vi "RUS Sweep -- write line to Temperatures file.vi"(4 "voltage":dbl, 6 "filename cluster OUT":T1={"mmddyy (str)"="", "counter (str)"="", "to F (kHz)"=0.0, "from F (kHz)"=0.0, "temperature (K)"=0.0, "date/time string"="", "time stamp"=timestamp(19856294.882018566 s since 1904-01-01), "base name"="", "temperature (str)"="", "from F (str)"="", "to F (str)"="", "format"=enum."no date string", "power (V)"=0.0, "power (str) "="", "Magn Field (T)"=0.0, "Magn Field (str)"=""}, 8 "error in":errorcluster, 9 "sweep folder path":path, 10 "file path":path, 11 "LTC Temperature":dbl) -> (0 "error out":errorcluster={"status"=TRUE, "code"=-200019, "source"="DAQmx Read (Analog 1D Wfm NChan NSamp).vi:1<append>\n<B>Task Name: </B>_unnamedTask<2C36>"})   [LabVIEW 2015]
uses:
  file -- scan filename.ctl
  ctl -- name dispatcher -- action.ctl
  file -- 9w path.vi
  <vilib>/Utility/file.llb/Write To Spreadsheet File (string).vi
  <vilib>/Utility/file.llb/Write To Spreadsheet File (DBL).vi
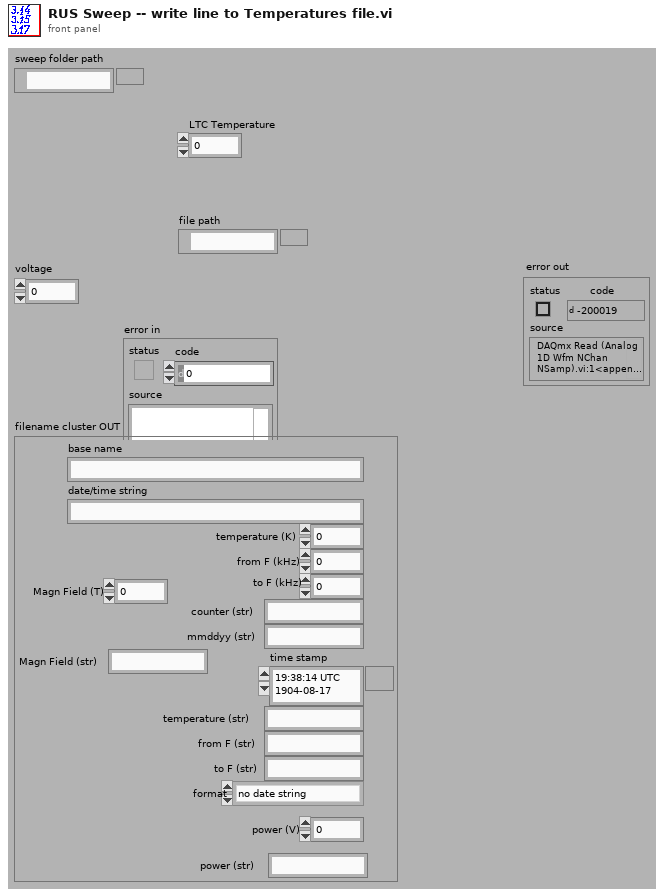
[diagram p1: front panel]
types:
  T1 = typedef "file -- scan filename.ctl" = cluster{"mmddyy (str)":string, "counter (str)":string, "to F (kHz)":dbl, "from F (kHz)":dbl, "temperature (K)":dbl, "date/time string":string, "time stamp":timestamp, "base name":string, "temperature (str)":string, "from F (str)":string, "to F (str)":string, "format":enum16{"no date string", "with date string"}, "power (V)":dbl, "power (str) ":string, "Magn Field (T)":dbl, "Magn Field (str)":string}
  T2 = typedef "ctl -- name dispatcher -- action.ctl" = enum16{"peak frequency", "peak frequency DUMP", "peak gamma DUMP", "peak gamma", "peak frequency TEST", "peak gamma TEST", "ultrasonic power", "time in gamma", "set temperature ", "set temperature timer", "peak default gamma", "last scan file", "peak freq gamma TEST", "peak NAMES", "errors", "P_I_D", "P", "I", "D", "power vs time", "power vs time TIMER", "void", "power log", "set temperature - SINE", "itc ltc log", "peak - time in gamma"}
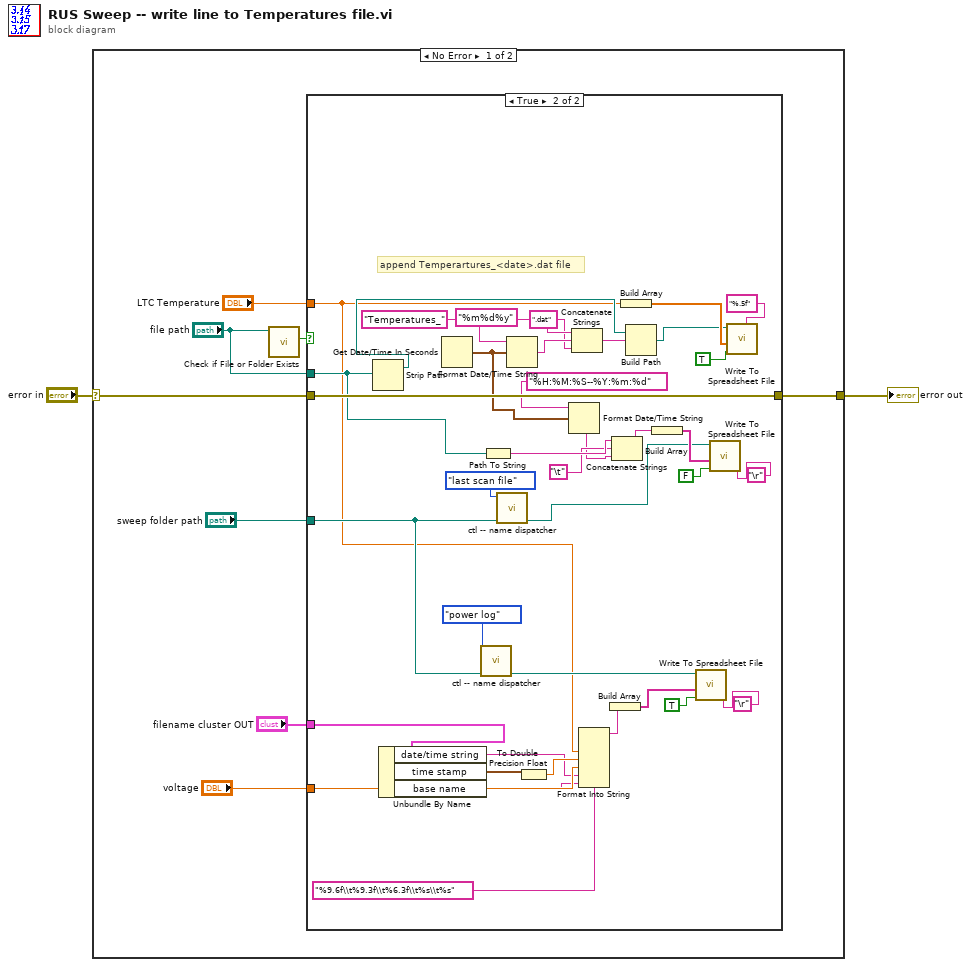
[diagram p0: block diagram]
diagram:
  n1 = case shown="No Error" "error in" {
    selector: "error in" -> [w6 w50]
    tunnel: [w7 w50] -> w2
    frame No Error {
      n2 = call <vilib>:"Check if File or Folder Exists.vi"("path"="file path") -> ("file or folder exists?"=w10:bool)  [unwired: 8 in, 2 out]
      n3 = case shown="True" w10 {
        tunnel: "file path" -> [_ w38]
        tunnel: "LTC Temperature" -> [_ w20]
        tunnel: w6 -> [w11 w40]
        tunnel: [w11 w40] -> w7
        tunnel: "sweep folder path" -> [_ w25]
        tunnel: "filename cluster OUT" -> [_ w18]
        tunnel: "voltage" -> [_ w17]
        frame False {
        }
        frame True {
          # "append Temperartures_<date>.dat file"
          n4 = Strip Path(path=w38) -> (stripped path=w39:path)  [unwired: 1 out]
          n5 = Unbundle By Name(w18) -> ("date/time string"=w15:string, "time stamp"=w21:timestamp, "base name"=w14:string)
          n6 = Get Date/Time In Seconds() -> (seconds since 1Jan1904=w37:timestamp)
          n7 = call "ctl -- name dispatcher.vi"("sweep folder path"=w25, "ctl name dispatch"=ctl_--_name_dispatcher_--_action."power log") -> ("file path"=w23:path)  [unwired: 7 in, 2 out]
          n8 = Path To String(path=w38) -> (string=w35:string)
          n9 = call "ctl -- name dispatcher.vi"("sweep folder path"=w25, "ctl name dispatch"=ctl_--_name_dispatcher_--_action."last scan file") -> ("file path"=w27:path)  [unwired: 7 in, 2 out]
          n10 = Format Date/Time String(time format string (%c)="%m%d%y", seconds (now)=w37) -> (date/time string=w48:string)  [unwired: 1 in]
          n11 = To Double Precision Float(number=w21) -> (double precision float=w16:dbl)
          n12 = Format Date/Time String(time format string (%c)="%H:%M:%S--%Y:%m:%d", seconds (now)=w37) -> (date/time string=w33:string)  [unwired: 1 in]
          n13 = Concatenate Strings("Temperatures_" ("string"), w48, ".dat" ("string")) -> (w46:string)
          n14 = Format Into String(format string="%9.6f\\t%9.3f\\t%6.3f\\t%s\\t%s", w20, w16, w17, w15, w14) -> (resulting string=w13:string)  [unwired: 2 in, 1 out]
          n15 = Build Array(w13) -> (w12:string[])
          n16 = Concatenate Strings(w35, "\t", w33) -> (w31:string)
          n17 = Build Array(w20) -> (w44:dbl[])
          n18 = Build Path(base path=w39, name or relative path=w46) -> (appended path=w43:path)
          n19 = Build Array(w31) -> (w30:string[])
          n20 = call-poly <vilib>:"Write To Spreadsheet File.vi"("delimiter (\\t)"="\r", "append to file? (new file:F)"=TRUE, "1D data"=w12, "file path (dialog if empty)"=w23) -> ()  [unwired: 4 in, 1 out]
          n21 = call-poly <vilib>:"Write To Spreadsheet File.vi"("delimiter (\\t)"="\r", "append to file? (new file:F)"=FALSE, "1D data"=w30, "file path (dialog if empty)"=w27) -> ()  [unwired: 4 in, 1 out]
          n22 = call-poly <vilib>:"Write To Spreadsheet File.vi"("format (%.3f)"="%.5f", "append to file? (new file:F)"=TRUE, "1D data"=w44, "file path (dialog if empty)"=w43) -> ()  [unwired: 4 in, 1 out]
        }
      }
    }
    frame Error {
    }
  }
  "error out" <- w2
